vi "GetConfigChain.vi"(8 "error in (no error)":errorcluster, 11 "reference in":refnum<class "Switch_MotorP5.lvclass">) -> (0 "error out":errorcluster, 2 "Config out":string[](array[string]), 3 "reference out":refnum<class "Switch_MotorP5.lvclass">)   [LabVIEW 2022 SP3, in "Switch_MotorP5.lvlib" / "Switch_MotorP5.lvclass"]
uses:
  Switch_MotorP5.lvclass
  Components/SwitchBase.lvlibp/SwitchBase.lvclass
  Components/ViPER.lvlibp/ViPER.lvclass
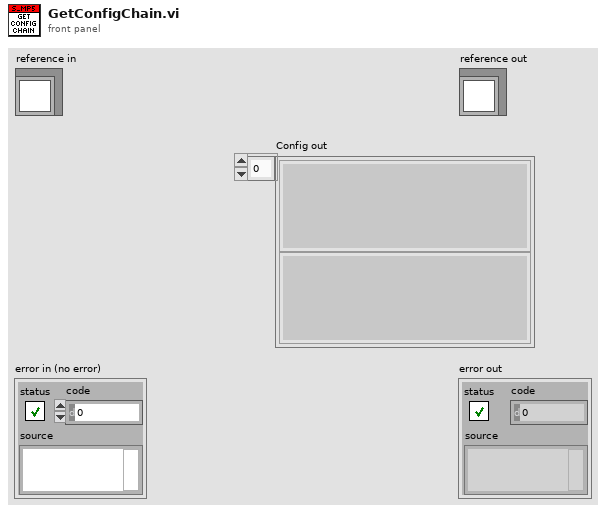
[diagram p1: front panel]
types:
  T1 = typedef "Switch_MotorP5.lvlib/Switch_MotorP5.lvclass/ObjectAttributes.ctl" = cluster{"Config":T2, "VISA":refnum<visa-resource-name>, "RPM":i32, "States":bool[], "UpdateEvent":refnum<user-event>, "Motor":enum32{"M1", "M2", "M3", "M4", "M5", "M6", "M7", "M8"}}
  T2 = typedef "Switch_MotorP5.lvlib/Switch_MotorP5.lvclass/Config.ctl" = cluster{"COM":refnum<visa-resource-name>, "SwitchMap":cluster{"Name":string, "Description":string, "Group":string, "IsGroup":bool, "Motor":enum32{"M1", "M2", "M3", "M4", "M5", "M6", "M7", "M8", "NA"}}[], "Sim":bool}
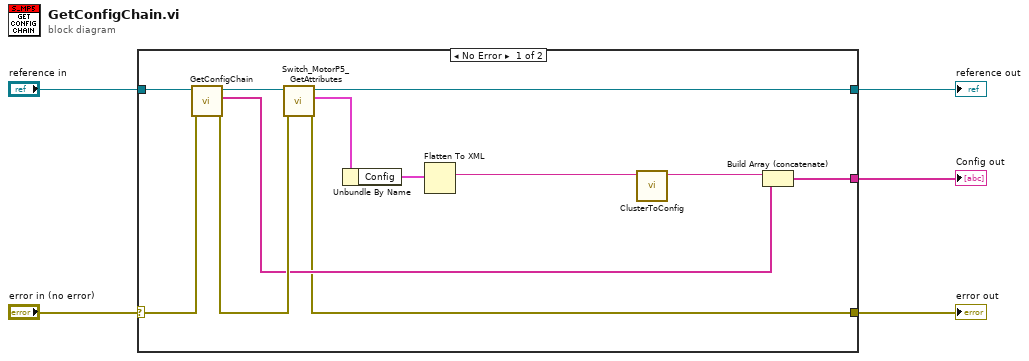
[diagram p0: block diagram]
diagram:
  n1 = case shown="No Error" "error in (no error)" {
    selector: "error in (no error)" -> [w13 w19]
    tunnel: [w6 w19] -> w4
    tunnel: [w11 w18] -> w2
    tunnel: "reference in" -> [w15 w18]
    tunnel: [w8 _] -> w1
    frame No Error {
      n2 = call-parent "GetConfigChain.vi"("error in (no error)"=w13, "reference in"=w15) -> ("error out"=w12:errorcluster, "Config out"=w9:string[], "reference out"=w14:refnum<class "Switch_MotorP5.lvclass">)  [unwired: 7 in]
      n3 = call "Switch_MotorP5_GetAttributes.vi"("error in (no error)"=w12, "reference in"=w14) -> ("error out"=w6:errorcluster, "Data"=w17:T1, "reference out"=w11:refnum<class "Switch_MotorP5.lvclass">)  [unwired: 6 in, 1 out]
      n4 = Unbundle By Name(w17) -> ("Config"=w16:T2)
      n5 = Flatten To XML(6:w16) -> (2:w7:string)
      n6 = call "ClusterToConfig.vi"("Cluster XML"=w7) -> ("Config XML"=w10:string)  [unwired: 10 in]
      n7 = Build Array (concatenate)(w10, w9) -> (w8:string[])
    }
    frame Error {
    }
  }
  "error out" <- w4
  "reference out" <- w2
  "Config out" <- w1
